vi "AI Comtinuous Engine Complete Testing.vi"   [LabVIEW 2009]
uses:
  Controls/SLL DE Virtual Chart Datalog Driver Options.ctl
  Controls/SLL DE Circular Buffer Options.ctl
  Controls/SLL DE Circular Buffer Pointers List.ctl
types:
  T1 = typedef "SLL DE Virtual Chart Datalog Driver Options.ctl" = enum16{"Initialise", "Write Headings", "Write", "Check File Size", "Read", "Clear"}
  T2 = typedef "SLL DE Circular Buffer Options.ctl" = enum16{"Initialize", "Init Pointer X", "Write", "Read Single Value", "Read Pointer X (Multi Value)", "Clear Data"}
  T3 = typedef "SLL DE Circular Buffer Pointers List.ctl" = enum16{"Graph Pointer", "File Log Pointer", "Pointer 3", "Pointer 4"}
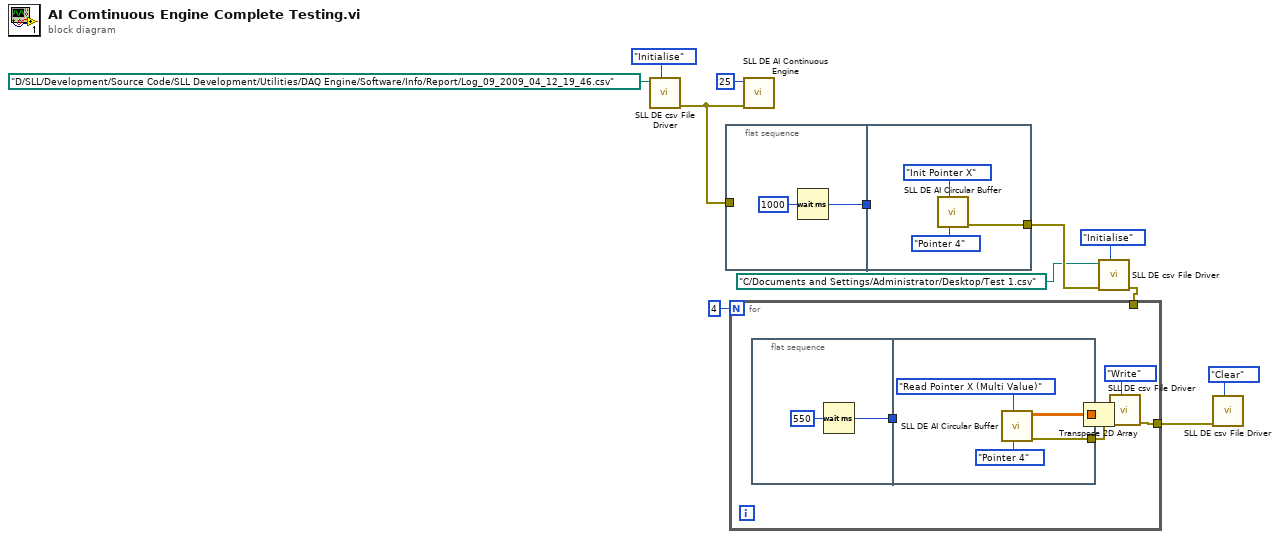
[diagram p0: block diagram]
diagram:
  n1 = call "SLL DE csv File Driver.vi"("Datalog Driver Cases"=SLL_DE_Virtual_Chart_Datalog_Driver_Options."Initialise", "Datalog path (use dialog)"=path "D:/SLL/Development/Source Code/SLL Development/Utilities/DAQ Engine/Software/Info/Report/Log_09_2009_04_12_19_46.csv") -> ("error out"=w9:errorcluster)  [unwired: 5 in, 4 out]
  n2 = flat-sequence {
    tunnel: w9 -> [_]
    tunnel: [w13] -> w8
    tunnel: w8 -> [_]
    tunnel: [w15] -> w5
    frame #0 {
      n3 = Wait (ms)(milliseconds to wait=u32 1000) -> (millisecond timer value=w13:u32)
    }
    frame #1 {
      n4 = call "SLL DE AI Circular Buffer.vi"("Pointers"=SLL_DE_Circular_Buffer_Pointers_List."Pointer 4", "Options"=SLL_DE_Circular_Buffer_Options."Init Pointer X") -> ("error Out"=w15:errorcluster)  [unwired: 4 in, 5 out]
    }
  }
  n5 = call "SLL DE AI Continuous Engine.vi"("error in (no error)"=w9, "Delay (ms)"=u32 25) -> ()  [unwired: 10 out]
  n6 = call "SLL DE csv File Driver.vi"("Datalog Driver Cases"=SLL_DE_Virtual_Chart_Datalog_Driver_Options."Initialise", "error in(no error)"=w5, "Datalog path (use dialog)"=path "C:/Documents and Settings/Administrator/Desktop/Test 1.csv") -> ("error out"=w4:errorcluster)  [unwired: 4 in, 4 out]
  n7 = for {
    N: 4 -> [_]
    tunnel: w4 -> [_]
    tunnel: [w20] -> w1
    n8 = flat-sequence {
      tunnel: [w24] -> w23
      tunnel: w23 -> [_]
      tunnel: [w27] -> w21
      tunnel: [w26] -> w19
      frame #0 {
        n9 = Wait (ms)(milliseconds to wait=u32 550) -> (millisecond timer value=w24:u32)
      }
      frame #1 {
        n10 = call "SLL DE AI Circular Buffer.vi"("Pointers"=SLL_DE_Circular_Buffer_Pointers_List."Pointer 4", "Options"=SLL_DE_Circular_Buffer_Options."Read Pointer X (Multi Value)") -> ("error Out"=w27:errorcluster, "Output Data"=w26:sgl[][])  [unwired: 4 in, 4 out]
      }
    }
    n11 = Transpose 2D Array(2D array=w19) -> (transposed array=w18:sgl[][])
    n12 = call "SLL DE csv File Driver.vi"("Datalog Driver Cases"=SLL_DE_Virtual_Chart_Datalog_Driver_Options."Write", "error in(no error)"=w21, "Data In"=w18) -> ("error out"=w20:errorcluster)  [unwired: 4 in, 4 out]
  }
  n13 = call "SLL DE csv File Driver.vi"("Datalog Driver Cases"=SLL_DE_Virtual_Chart_Datalog_Driver_Options."Clear", "error in(no error)"=w1) -> ()  [unwired: 5 in, 5 out]
